vi "Init.vi"(8 "error in (no error)":errorcluster, 9 "Server (Client)":bool, 10 "VectoInfo":refnum<class "VectoInfo.lvclass">) -> (0 "error out":errorcluster, 3 "VectoTCPConnectionHandler out":refnum<class "VectoTCPConnectionHandler.lvclass">)   [LabVIEW 2020, in "Vecto.lvlib" / "VectoTCPConnectionHandler.lvclass"]
uses:
  VectoTCPConnectionHandler.lvclass
  VectoService/VectoInfo.lvclass
  VectoTCPConnectionHandler.lvclass/VectoTCPConnectionHandler.ctl
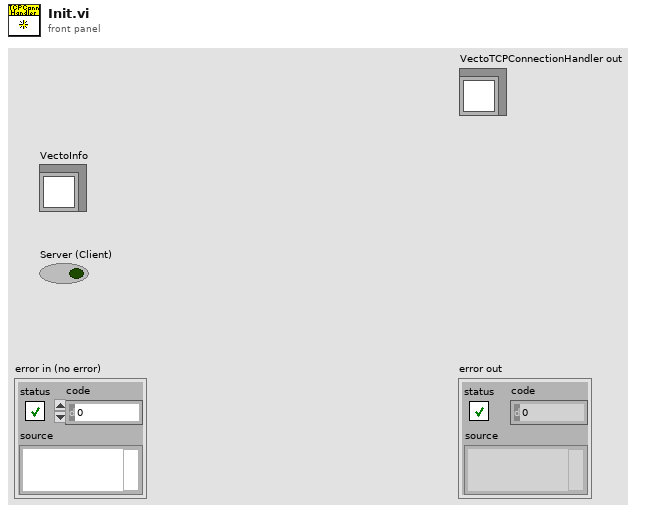
[diagram p1: front panel]
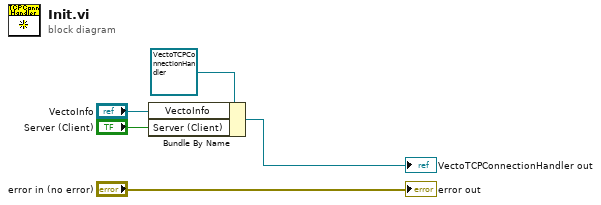
[diagram p0: block diagram]
diagram:
  n1 = Bundle By Name(cluster=refnum<class "VectoTCPConnectionHandler.lvclass"> refnum ("VectoTCPConnectionHandler in"), "VectoInfo"="VectoInfo", "Server (Client)"="Server (Client)") -> (→"VectoTCPConnectionHandler out":refnum<class "VectoTCPConnectionHandler.lvclass">)
  "error out" <- "error in (no error)"
